vi "Vision Processing.vi"(4 "error in (no error)":errorcluster, 7 "Image Size":T2=enum."320x240") -> ()   [LabVIEW 2016]
doc: "This VI runs in parallel to other tasks. It gets images from the camera, processes them for color or shape and use that information to affect robot behavior."
uses:
  <vilib>/Rock Robotics/WPI/Camera/WPI_CameraImageSize.ctl
  <vilib>/Rock Robotics/WPI/SPI/WPI_SPIMode.ctl
  <vilib>/Rock Robotics/SystemInterfaces/spilib/spi_bus.ctl
  Global Frame Data.vi
  Robot Global Data.vi
  <vilib>/Rock Robotics/WPI/Camera/WPI_CameraWhite Balance Values.ctl
  <vilib>/Rock Robotics/WPI/Camera/WPI_CameraExposure Values.ctl
  <vilib>/Rock Robotics/WPI/Camera/WPI_CameraFrameRate.ctl
  Frame Data.vi
panel:
  out "2D Picture":picture
  in  "Sample Size":dbl
  out "Complete frames per second":dbl
  out "Completed?":bool
  out "Objects Found":u16
  out "Frame Data":T1(array[cluster])
  out "Most Recent Frame":u8[](array[numeric]) format="%x"
  out "Times Run":i32
  out "Decimal Data":u8[](array[numeric])
  out "Average Loop Rate":dbl
  out "Hexadecimal Data":u8[](array[numeric]) format="%x"
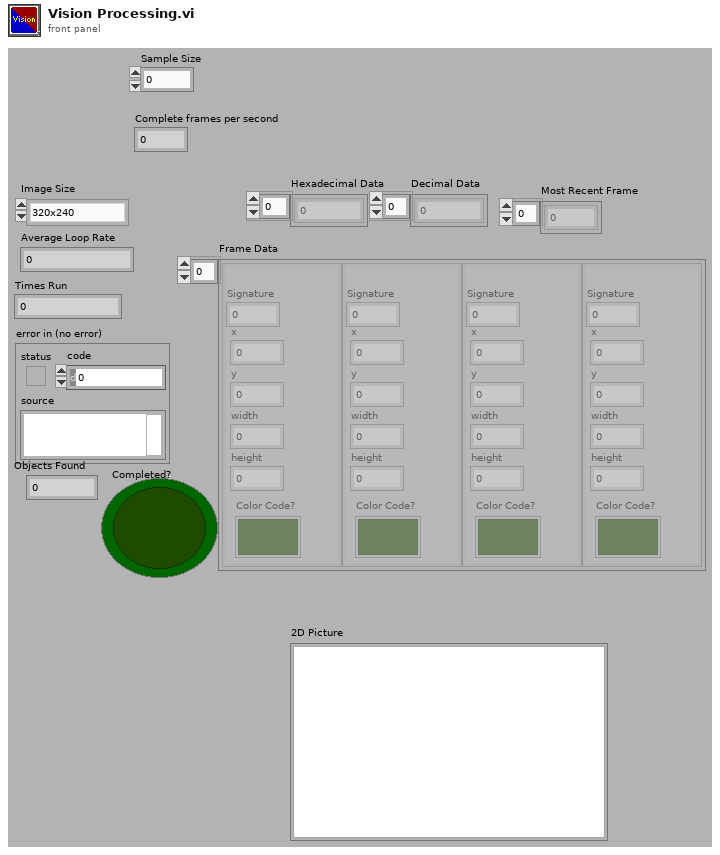
[diagram p1: front panel]
types:
  T1 = cluster{"x":u16, "y":u16, "width":u16, "height":u16, "Signature":u16, "Color Code?":bool}[]
  T2 = typedef "WPI_CameraImageSize.ctl" = enum16{"640x480", "320x240", "160x120", "Custom"}
  T3 = typedef "spi_bus.ctl" = enum16{"SPI On-Board, CS0", "SPI On-Board, CS1", "SPI On-Board, CS2", "SPI On-Board, CS3", "SPI MXP", "Invalid"}
  T4 = typedef "WPI_SPIMode.ctl" = enum16{"Mode 0 (Clk Idle Low,Sample on Leading)", "Mode 1 (Clk Idle Low,Sample on Trailing)", "Mode 2 (Clk Idle High,Sample on Leading)", "Mode 3 (Clk Idle High,Sample on Trailing)"}
  T5 = typedef "WPI_SPIDevRef.ctl" = cluster{"DevStatus":errorcluster, "Handle":i32, "SPI Bus":T3}
  T6 = cluster{"left":i16, "top":i16, "right":i16, "bottom":i16}
  T7 = typedef "WPI_CameraFrameRate.ctl" = u32
  T8 = typedef "WPI_CameraExposure Values.ctl" = enum16{"Auto", "Flicker-free 50 Hz", "Flicker-free 60 Hz", "Hold current", "Custom"}
  T9 = typedef "WPI_CameraWhite Balance Values.ctl" = enum16{"Auto", "Fixed indoor", "Fixed outdoor 1", "Fixed outdoor 2", "Fixed fluorescent 1", "Fixed fluorescent 2", "Hold current", "Custom"}
  T10 = typedef "Image Type" = u32
  T11 = typedef "WPI_CameraDevRef.ctl" = cluster{"Camera Address":string, "CameraStatus":errorcluster}
  T12 = typedef "IMAQ Image.ctl" = refnum<image>
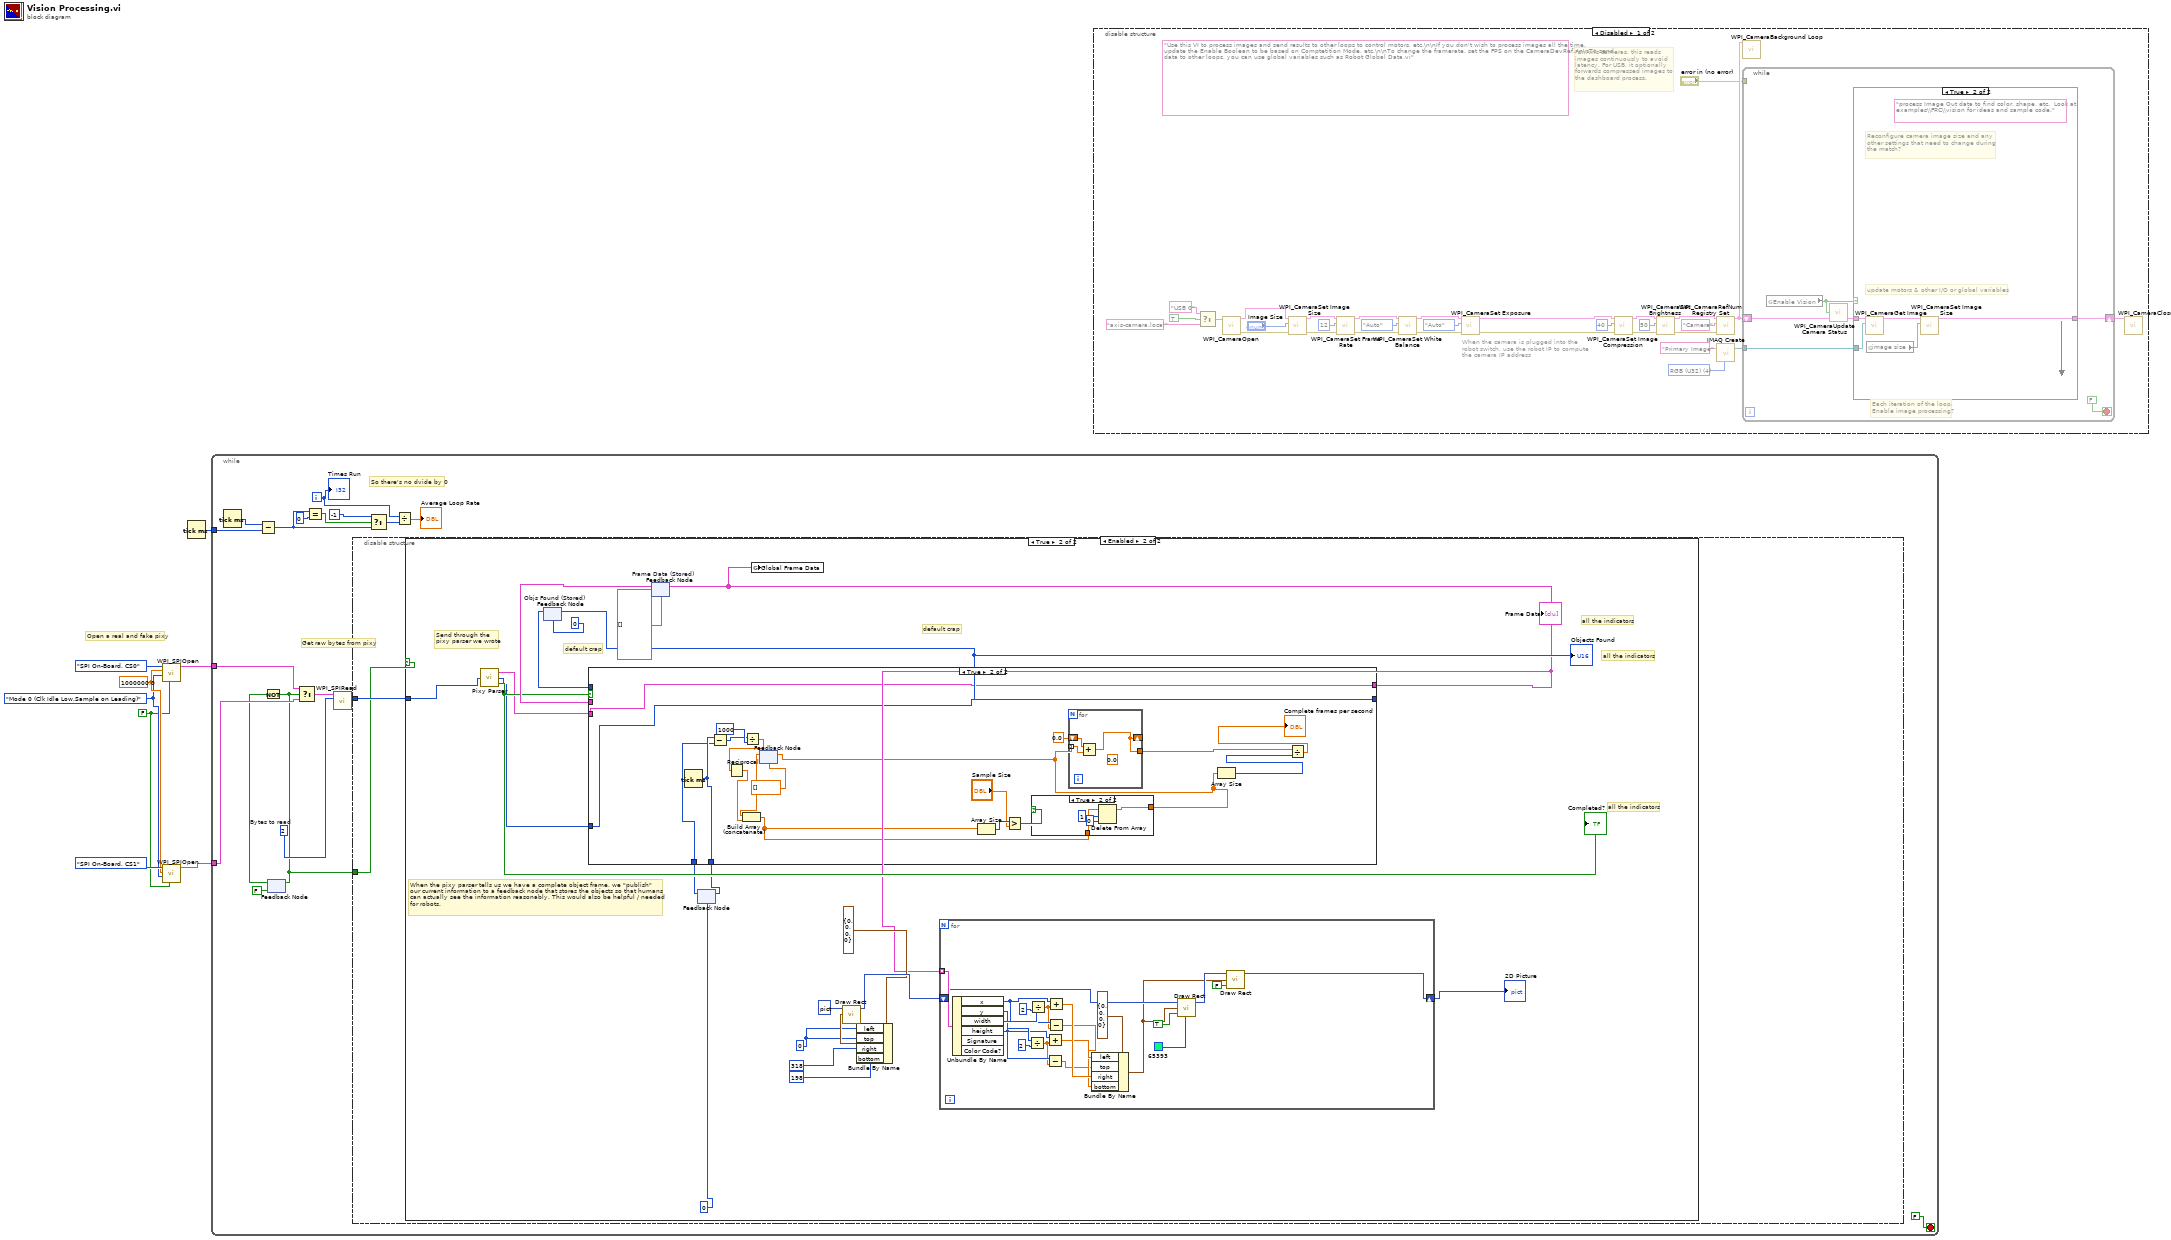
[diagram p0: block diagram]
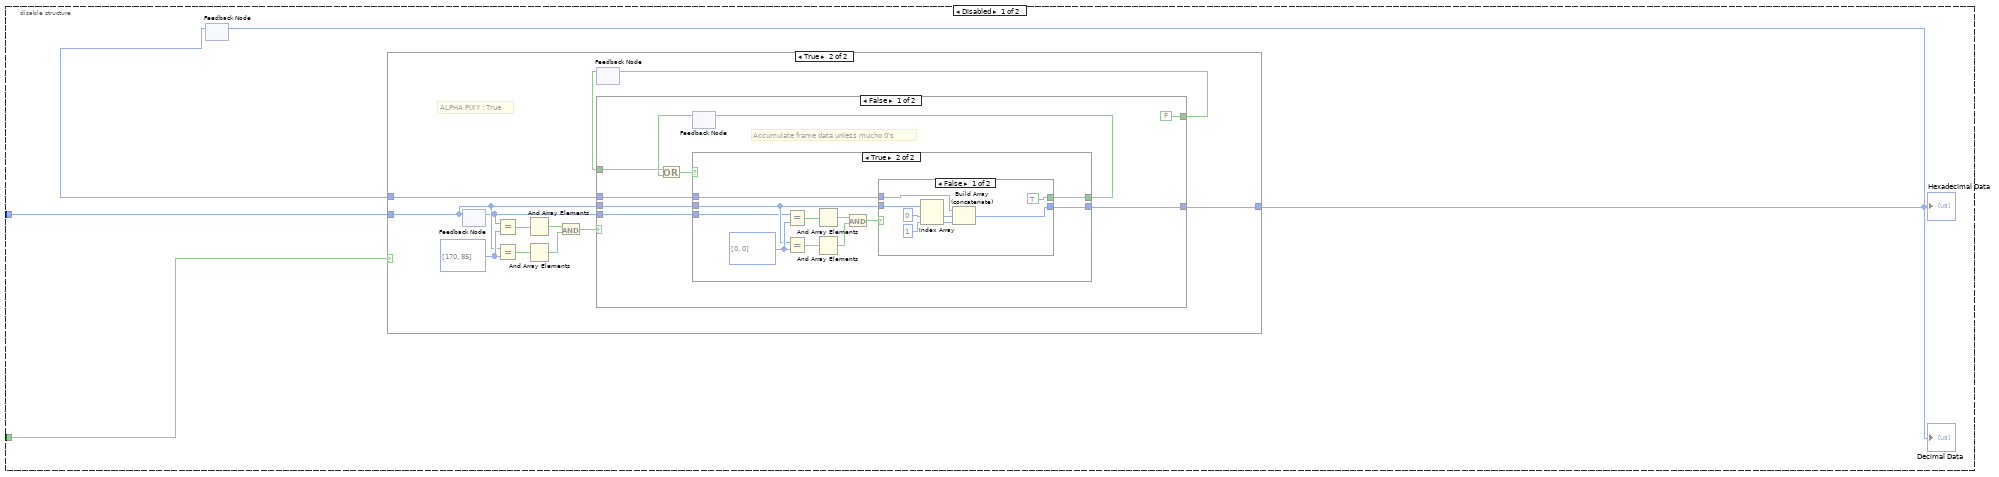
[diagram p2: hidden frame]
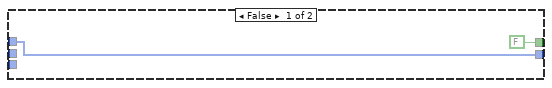
[diagram p4: hidden frame]
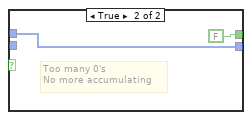
[diagram p5: hidden frame]
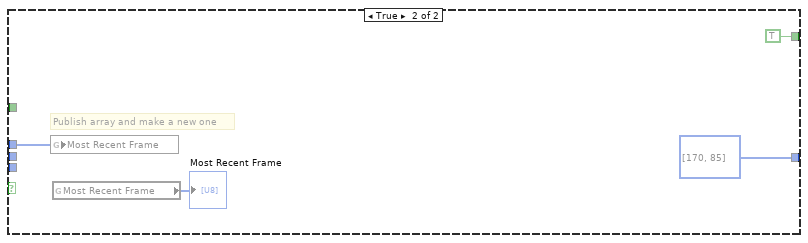
[diagram p6: hidden frame]
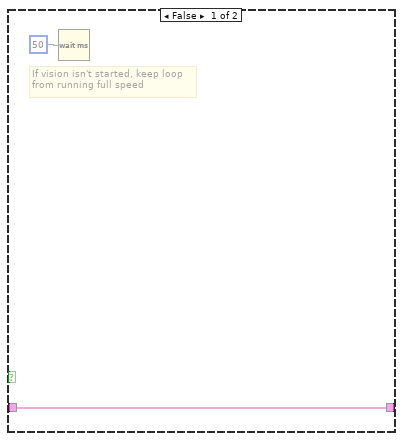
[diagram p10: hidden frame]
diagram:
  w4 = 1000000.0 ("Clock Rate (Hz)")
  w3 = WPI_SPIMode."Mode 0 (Clk Idle Low,Sample on Leading)" ("Mode (3)")
  w2 = FALSE ("Chip Select Active High (F)")
  # "Open a real and fake pixy"
  n1 = call <vilib>:"WPI_SPIOpen.vi"("Chip Select Active High (F)"=w2, "Mode (3)"=w3, "Clock Rate (Hz)"=w4, "SPI Bus"=spi_bus."SPI On-Board, CS0") -> ("SPIDevRef"=w7:T5)  [unwired: 6 in, 1 out]
  n2 = call <vilib>:"WPI_SPIOpen.vi"("Chip Select Active High (F)"=w2, "Mode (3)"=w3, "Clock Rate (Hz)"=w4, "SPI Bus"=spi_bus."SPI On-Board, CS1") -> ("SPIDevRef"=w1:T5)  [unwired: 6 in, 1 out]
  n3 = Tick Count (ms)() -> (millisecond timer value=w6:u32)
  n4 = while {
    tunnel: w7 -> [w16]
    tunnel: w6 -> [w9]
    tunnel: w1 -> [w15]
    i -> [w24]
    stop <- FALSE stop-if-true
    w17 = 2  # Bytes to read
    # "Get raw bytes from pixy"
    # "So there's no dvide by 0"
    n5 = Tick Count (ms)() -> (millisecond timer value=w25:u32)
    n6 = Subtract(x=w25, y=w9) -> (x-y=w18:u32)
    n7 = feedback #1(FALSE) -> (w12:bool)
    n8 = Not(x=w12) -> (.not. x?=w10:bool)
    n9 = feedback-in #1(w10) -> ()
    n10 = Select(t=w16, s=w10, f=w15) -> (s? t:f=w14:T5)
    n11 = Equal?(x=w18, y=u32 0) -> (x = y?=w21:bool)
    n12 = call <vilib>:"WPI_SPIRead.vi"("Num to Read"=w17, "SPIDevRef"=w14) -> ("Received Data"=w11:u8[])  [unwired: 7 in, 2 out]
    n13 = disable-structure shown="Enabled" {
      disable-tunnel: w11 -> [w30 w81]
      disable-tunnel: w10 -> [w29 w80]
      frame Disabled {
        n14 = feedback #2() -> (w28:u8[])  [unwired: 1 in]
        n15 = case shown="True" w29 {
          tunnel: w30 -> [_ w37]
          tunnel: w28 -> [w31 w36]
          tunnel: [w31 w35] -> w27
          frame False {
            # "IMPOSTER PIXY : False"
          }
          frame True {
            w43 = u8[] [170, 85]
            # "ALPHA PIXY : True"
            n16 = feedback-in #3(w37) -> ()
            n17 = feedback #3() -> (w34:u8[])  [unwired: 1 in]
            n18 = Equal?(x=w34, y=w43) -> (x = y?=w41:bool[])
            n19 = Equal?(x=w37, y=w43) -> (x = y?=w42:bool[])
            n20 = And Array Elements(Boolean array=w41) -> (logical AND=w40:bool)
            n21 = And Array Elements(Boolean array=w42) -> (logical AND=w39:bool)
            n22 = And(x=w40, y=w39) -> (x .and. y?=w38:bool)
            n23 = feedback #4() -> (w32:bool)  [unwired: 1 in]
            n24 = case shown="False" w38 {
              tunnel: w37 -> [w50 _]
              tunnel: w36 -> [w52 w78]
              tunnel: [w51 u8[] [170, 85]] -> w35
              tunnel: w34 -> [w49 _]
              tunnel: [FALSE TRUE] -> w33
              tunnel: w32 -> [w47 _]
              frame False {
                # "Accumulate frame data unless mucho 0's"
                n25 = feedback #5() -> (w46:bool)  [unwired: 1 in]
                n26 = Or(x=w47, y=w46) -> (x .or. y?=w45:bool)
                n27 = case shown="True" w45 {
                  tunnel: w52 -> [w54 w65]
                  tunnel: [w54 w64] -> w51
                  tunnel: w50 -> [_ w59]
                  tunnel: w49 -> [_ w58]
                  tunnel: [FALSE w55] -> w48
                  frame False {
                  }
                  frame True {
                    w60 = u8[] [0, 0]
                    n28 = Equal?(x=w58, y=w60) -> (x = y?=w62:bool[])
                    n29 = Equal?(x=w59, y=w60) -> (x = y?=w61:bool[])
                    n30 = And Array Elements(Boolean array=w62) -> (logical AND=w57:bool)
                    n31 = And Array Elements(Boolean array=w61) -> (logical AND=w63:bool)
                    n32 = And(x=w57, y=w63) -> (x .and. y?=w56:bool)
                    n33 = case shown="False" w56 {
                      tunnel: w59 -> [w69 _]
                      tunnel: w65 -> [w68 w75]
                      tunnel: [w67 w75] -> w64
                      tunnel: [TRUE FALSE] -> w55
                      frame False {
                        n34 = Index Array(array=w69, index #1=0 ("index"), index #2=1 ("index")) -> (element #1=w72:u8, element #2=w73:u8)
                        n35 = Build Array (concatenate)(w68, w72, w73) -> (w67:u8[])
                      }
                      frame True {
                        # "Too many 0's\nNo more accumulating"
                      }
                    }
                  }
                }
                n36 = feedback-in #5(w48) -> ()
              }
              frame True {
                # "Publish array and make a new one"
                n37 = global write "Frame Data.vi" "Most Recent Frame"(w78) -> ()
                n38 = global read "Frame Data.vi" "Most Recent Frame"() -> (→"Most Recent Frame":u8[])
              }
            }
            n39 = feedback-in #4(w33) -> ()
          }
        }
        "Hexadecimal Data" <- w27
        "Decimal Data" <- w27
        n40 = feedback-in #2(w27) -> ()
      }
      frame Enabled {
        n41 = case shown="True" w80 {
          tunnel: w81 -> [_ w102]
          frame False {
            # "nothing happens because its fake"
          }
          frame True {
            w85 = i16 0 ("left")
            # "default crap"
            # "all the indicators"
            # "all the indicators"
            # "all the indicators"
            # "default crap"
            # "When the pixy parser tells us we have a complete object frame, we \"publish\"\nour current information to a feedback node that stores the objects so that humans\ncan actually see the information reasonably. This would also be helpful / needed\nfor robots."
            # "Send through the\npixy parser we wrote"
            n42 = call "Pixy Parser.vi"("Array"=w102) -> ("Array 2"=w98:T1, "Objects Found"=w97:u16, "Completed?"=w99:bool)
            "Completed?" <- w99
            n43 = feedback #6 "Objs Found (Stored)"(u16 0 ("Objects Found")) -> (w101:u16)
            n44 = feedback #7 "Frame Data (Stored)"(T1 [] ("Array 2")) -> (w100:T1)
            n45 = feedback #8(u32 0) -> (w93:u32)
            n46 = case shown="True" w99 {
              tunnel: w101 -> [w125 _]
              tunnel: w100 -> [w126 _]
              tunnel: [w126 w127] -> w82
              tunnel: [w125 w145] -> w94
              tunnel: w98 -> [_ w127]
              tunnel: w97 -> [_ w145]
              tunnel: w93 -> [w124 w143]
              tunnel: [w124 w144] -> w91
              frame False {
              }
              frame True {
                n47 = Tick Count (ms)() -> (millisecond timer value=w144:u32)
                n48 = Subtract(x=w144, y=w143) -> (x-y=w141:u32)
                n49 = Divide(x=w141, y=u32 1000) -> (x/y=w140:dbl)
                n50 = Reciprocal(x=w140) -> (1/x=w130:dbl)
                n51 = feedback #9(dbl[] []) -> (w131:dbl[])
                n52 = Build Array (concatenate)(w131, w130) -> (w128:dbl[])
                n53 = Array Size(array=w128) -> (size(s)=w138:i32)
                n54 = Greater?(x=w138, y="Sample Size") -> (0:w136:bool)
                n55 = case shown="True" w136 {
                  tunnel: w128 -> [w149 w153]
                  tunnel: [w149 w150] -> w132
                  frame False {
                  }
                  frame True {
                    n56 = Delete From Array(array=w153, length=1, index=0) -> (array with subset deleted=w150:dbl[])  [unwired: 1 out]
                  }
                }
                n57 = feedback-in #9(w132) -> ()
                n58 = for {
                  tunnel: w132 -> [w148] mode=indexing
                  tunnel: [w146] -> w135
                  shift-right: [w146] -> _
                  shift-left: 0.0 -> [w147]
                  (unwired) 0.0
                  n59 = Add(x=w147, y=w148) -> (x+y=w146:dbl)
                }
                n60 = Array Size(array=w132) -> (size(s)=w134:i32)
                n61 = Divide(x=w135, y=w134) -> (x/y=→"Complete frames per second":dbl)
              }
            }
            "Frame Data" <- w82
            "Objects Found" <- w94
            n62 = feedback-in #6(w94) -> ()
            n63 = feedback-in #7(w82) -> ()
            n64 = feedback-in #8(w91) -> ()
            n65 = global write "Global Frame Data.vi" "Global Frame Data"(w82) -> ()
            n66 = Bundle By Name(cluster=T6 {"left"=0, "top"=0, "right"=0, "bottom"=0} ("rect"), "left"=w85, "top"=w85, "right"=i16 318, "bottom"=i16 198) -> (w88:T6)
            n67 = call <vilib>:"Draw Rect.vi"("picture"=picture data[5B], "rect"=w88) -> ("new picture"=w90:picture)  [unwired: 7 in]
            n68 = for {
              tunnel: w82 -> [w123] mode=indexing
              shift-right: [w103] -> w83
              shift-left: w90 -> [w107]
              n69 = Unbundle By Name(w123) -> ("x"=w114:u16, "y"=w110:u16, "width"=w119:u16, "height"=w115:u16)  [unwired: 2 out]
              n70 = Divide(x=w115, y=u16 2) -> (x/y=w109:dbl)
              n71 = Divide(x=w119, y=u16 2) -> (x/y=w113:dbl)
              n72 = Add(x=w110, y=w109) -> (x+y=w111:dbl)
              n73 = Subtract(x=w110, y=w109) -> (x-y=w108:dbl)
              n74 = Add(x=w114, y=w113) -> (x+y=w118:dbl)
              n75 = Subtract(x=w114, y=w113) -> (x-y=w112:dbl)
              n76 = Bundle By Name(cluster=T6 {"left"=0, "top"=0, "right"=0, "bottom"=0} ("rect"), "left"=w112, "top"=w108, "right"=w118, "bottom"=w111) -> (w105:T6)
              n77 = call <vilib>:"Draw Rect.vi"("picture"=w107, "rect"=w105, "fill?(F)"=TRUE, "color(black)"=u32 65393) -> ("new picture"=w106:picture)  [unwired: 5 in]
              n78 = call <vilib>:"Draw Rect.vi"("picture"=w106, "rect"=w105, "fill?(F)"=FALSE) -> ("new picture"=w103:picture)  [unwired: 6 in]
            }
            "2D Picture" <- w83
          }
        }
      }
    }
    n79 = Select(t=-1, s=w21, f=w18) -> (s? t:f=w20:u32)
    n80 = Divide(x=w24, y=w20) -> (x/y=→"Average Loop Rate":dbl)
    "Times Run" <- w24
  }
  n81 = disable-structure shown="Disabled" {
    frame Disabled {
      (unwired) "Use this VI to process images and send results to other loops to control motors, etc.\n\nIf you don't wish to process images all the time, update the Enable Boolean to be based on Comptetition Mode, etc.\n\nTo change the framerate, set the FPS on the CameraDevRef..\n\nTo send data to other loops, you can use global variables such as Robot Global Data.vi"
      w184 = T10 4 items=["Grayscale (U8)", "Grayscale (I16)", "Grayscale (SGL)", "Complex (CSG)", "RGB (U32)", "HSL (U32)", "RGB (U64)"] ("Image Type")
      # "When the camera is plugged into the\nrobot switch, use the robot IP to compute\nthe camera IP address"
      # "For Axis cameras, this reads\nimages continuously to avoid\nlatency. For USB, it optionally\nforwards compressed images to\nthe dashboard process."
      n82 = Select(t="USB 0" ("format string"), s=TRUE ("dot notation? (F)"), f="axis-camera.local" ("format string")) -> (s? t:f=w155:string)
      n83 = call <vilib>:"WPI_CameraOpen.vi"("Camera Address"=w155) -> ("error out"=w172:errorcluster, "CameraDevRef"=w173:T11)  [unwired: 1 in, 8 out]
      n84 = call <vilib>:"WPI_CameraSet Image Size.vi"("error in (no error)"=w172, "Image Size"="Image Size", "CameraDevRef"=w173) -> ("error out"=w171:errorcluster, "CameraDevRef Out"=w174:T11)  [unwired: 1 in, 6 out]
      n85 = call <vilib>:"WPI_CameraSet Frame Rate.vi"("error in (no error)"=w171, "Frame Rate (fps)"=T7 12, "CameraDevRef"=w174) -> ("error out"=w170:errorcluster, "CameraDevRef Out"=w176:T11)  [unwired: 7 out]
      n86 = call <vilib>:"WPI_CameraSet White Balance.vi"("error in (no error)"=w170, "White Balance"=WPI_CameraWhite_Balance_Values."Auto", "CameraDevRef"=w176) -> ("error out"=w169:errorcluster, "CameraDevRef Out"=w175:T11)  [unwired: 1 in, 6 out]
      n87 = call <vilib>:"WPI_CameraSet Exposure.vi"("error in (no error)"=w169, "Exposure"=WPI_CameraExposure_Values."Auto", "CameraDevRef"=w175) -> ("error out"=w168:errorcluster, "CameraDevRef Out"=w178:T11)  [unwired: 1 in, 6 out]
      n88 = call <vilib>:"WPI_CameraSet Image Compression.vi"("error in (no error)"=w168, "Compression"=40, "CameraDevRef"=w178) -> ("error out"=w167:errorcluster, "CameraDevRef Out"=w177:T11)  [unwired: 7 out]
      n89 = call <vilib>:"WPI_CameraSet Brightness.vi"("error in (no error)"=w167, "Brightness"=50, "CameraDevRef"=w177) -> ("error out"=w165:errorcluster, "CameraDevRef Out"=w166:T11)  [unwired: 7 out]
      n90 = call <vilib>:"WPI_CameraRefNum Registry Set.vi"("error in (no error)"=w165, "refnum name"="Camera", "CameraDevRef"=w166) -> ("CameraDevRef"=w161:T11)  [unwired: 1 in, 7 out]
      n91 = call "IMAQ Create"("Image Name"="Primary Image", "Image Type"=w184) -> ("New Image"=w182:T12)  [unwired: 2 in, 2 out]
      n92 = call <vilib>:"WPI_CameraBackground Loop.vi"("CameraDevRef"=w161) -> ()  [unwired: 11 in]
      n93 = while {
        shift-right: [w189] -> w159
        shift-left: w161 -> [w187]
        tunnel: w182 -> [w188]
        tunnel: "error in (no error)" -> [_]
        stop <- FALSE stop-if-true
        # "Each iteration of the loop,\nEnable image processing?"
        n94 = global read "Robot Global Data.vi" "Enable Vision"() -> (w185:bool)
        n95 = call <vilib>:"WPI_CameraUpdate Camera Status.vi"("CameraDevRef In"=w187, "Enable Vision"=w185) -> ("CameraDevRef Out"=w186:T11)  [unwired: 3 in]
        n96 = case shown="True" w185 {
          tunnel: w188 -> [_ w196]
          tunnel: [w192 w197] -> w189
          tunnel: w186 -> [w192 w194]
          frame False {
            # "If vision isn't started, keep loop\nfrom running full speed"
            n97 = Wait (ms)(milliseconds to wait=u32 50) -> ()  [unwired: 1 out]
          }
          frame True {
            (unwired) "process Image Out data to find color, shape, etc.  Look at examples\\FRC\\vision for ideas and sample code."
            # "update motors & other I/O or global variables"
            # "Reconfigure camera image size and any\nother settings that need to change during\nthe match?"
            n98 = call <vilib>:"WPI_CameraGet Image.vi"("Image"=w196, "CameraDevRef"=w194) -> ("CameraDevRef Out"=w193:T11)  [unwired: 1 in, 8 out]
            n99 = global read "Robot Global Data.vi" "image size"() -> (w195:T2)
            n100 = call <vilib>:"WPI_CameraSet Image Size.vi"("Image Size"=w195, "CameraDevRef"=w193) -> ("CameraDevRef Out"=w197:T11)  [unwired: 2 in, 7 out]
          }
        }
      }
      n101 = call <vilib>:"WPI_CameraClose.vi"("CameraDevRef"=w159) -> ()  [unwired: 1 in, 10 out]
    }
    frame Enabled {
    }
  }
